vi "json_cache_ids.vi"(8 "error in (no error)":errorcluster) -> (0 "error out":errorcluster, 3 "cache ids":u64[](array[numeric]))   [LabVIEW 2017]
uses:
  json_element.ctl
  json_element_type.ctl
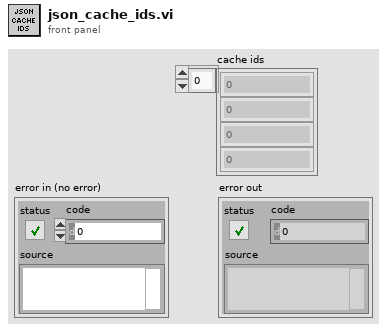
[diagram p1: front panel]
types:
  T1 = typedef "json_element.ctl" = cluster{"path":string, "type":T2, "value":variant}
  T2 = typedef "json_element_type.ctl" = enum8{"null", "bool", "int", "uint", "float", "string", "array", "object"}
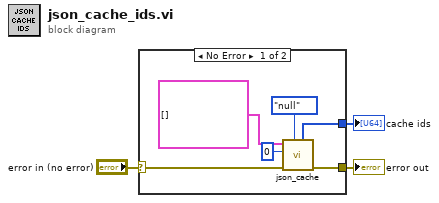
[diagram p0: block diagram]
diagram:
  n1 = case shown="No Error" "error in (no error)" {
    selector: "error in (no error)" -> [w9 w10]
    tunnel: [w5 _] -> w2
    tunnel: [w4 w10] -> w1
    frame No Error {
      n2 = call "json_cache.vi"("action"=enum8{"null", "get", "create", "delete"}."null", "error in (no error)"=w9, "cache id in"=u64 0, "elements in"=T1[] []) -> ("error out"=w4:errorcluster, "cache ids"=w5:u64[])  [unwired: 3 in, 3 out]
    }
    frame Error {
    }
  }
  "error out" <- w1
  "cache ids" <- w2
